vi "Add Default Free.vi"(8 "error in (no error)":errorcluster, 10 "ToModBus":bool, 11 "RTD in":refnum<class "RTD.lvclass">) -> (0 "error out":errorcluster, 3 "RTD out":refnum<class "RTD.lvclass">)   [LabVIEW 2012, in "Measurement Channels.lvlib" / "RTD.lvclass"]
uses:
  RTD.lvclass
  Class Channel/Channel.lvclass
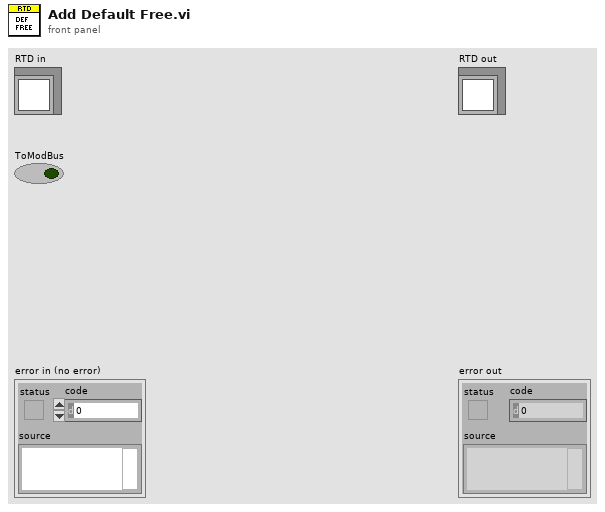
[diagram p1: front panel]
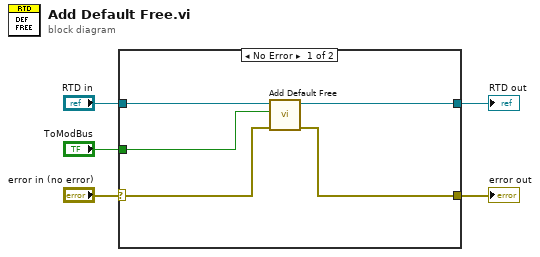
[diagram p0: block diagram]
diagram:
  n1 = case shown="No Error" "error in (no error)" {
    selector: "error in (no error)" -> [w6 w11]
    tunnel: [w10 w11] -> w5
    tunnel: [w9 w12] -> w4
    tunnel: "ToModBus" -> [w8 _]
    tunnel: "RTD in" -> [w7 w12]
    frame No Error {
      n2 = call-parent "Add Default Free.vi"("error in (no error)"=w6, "ToModBus"=w8, "Channel in"=w7) -> ("error out"=w10:errorcluster, "Channel out"=w9:refnum<class "RTD.lvclass">)  [unwired: 7 in]
    }
    frame Error {
    }
  }
  "error out" <- w5
  "RTD out" <- w4
